vi "Flatten to String.vi"(8 "error in (no error)":errorcluster, 9 "priority":i32, 10 "Message":refnum<class "Message.lvclass">, 11 "Flattener in":refnum<class "Message Flattener.lvclass">) -> (0 "error out":errorcluster, 2 "Flattened String":string, 3 "Flattener out":refnum<class "Message Flattener.lvclass">)   [LabVIEW 2020, in "Message Flattener.lvclass"]
doc: "This method uses the Flatten to String function to flatten a message object to a string that can be sent across the network. Override this method to implement a different serialization scheme."
uses:
  Message Flattener.lvclass
  <vilib>/ActorFramework/Message/Message.lvclass
  Message Flattener.lvclass/Message Flattener.ctl
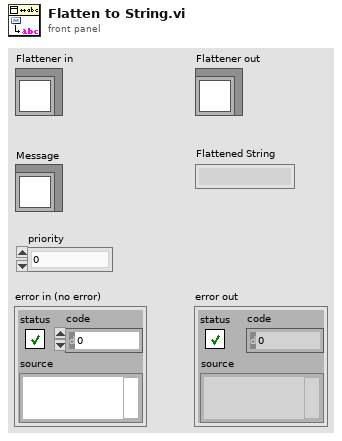
[diagram p1: front panel]
types:
  T1 = cluster{"Message":refnum<class "Message.lvclass">, "priority":i32}
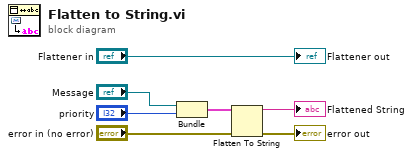
[diagram p0: block diagram]
diagram:
  n1 = Bundle("Message"="Message", "priority"="priority") -> (w6:T1)  [unwired: 1 in]
  n2 = Flatten To String(anything=w6, error in (no error)="error in (no error)") -> (data string=→"Flattened String":string, error out=→"error out":errorcluster)  [unwired: 2 in, 1 out]
  "Flattener out" <- "Flattener in"
